vi "Save PID to DB.vi"(8 "error in":errorcluster, 10 "PID":T1, 11 "Name":string) -> (0 "error out":errorcluster)   [LabVIEW 2016]
uses:
  PID Settings.ctl
  <vilib>/Rock Robotics/Network Tables/NT Write Numeric Array.vi
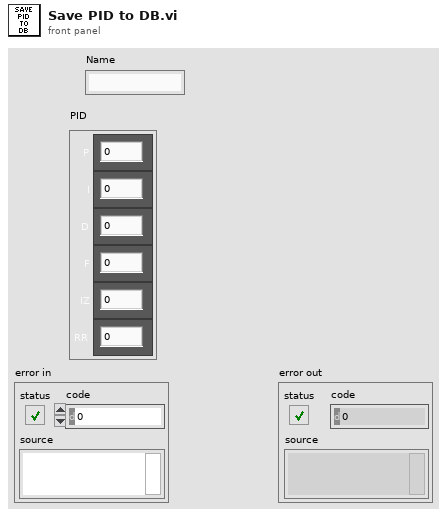
[diagram p1: front panel]
types:
  T1 = typedef "PID Settings.ctl" = cluster{"D":dbl, "F":dbl, "RR":dbl, "IZ":dbl, "P":dbl, "I":dbl}
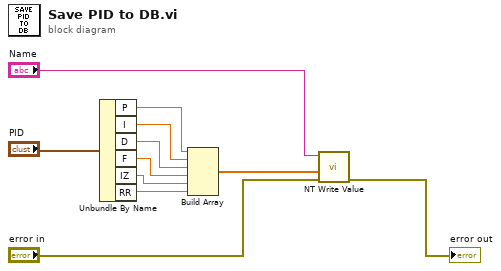
[diagram p0: block diagram]
diagram:
  n1 = Unbundle By Name("PID") -> ("P"=w10:dbl, "I"=w9:dbl, "D"=w8:dbl, "F"=w7:dbl, "IZ"=w6:dbl, "RR"=w5:dbl)
  n2 = Build Array(w10, w9, w8, w7, w6, w5) -> (w3:dbl[])
  n3 = call-poly <vilib>:"NT Write Value.vi"("error in"="error in", "Numeric Array"=w3, "Name"="Name") -> ("error out"=→"error out":errorcluster)  [unwired: 8 in]
